vi "Agilent ENA Series Receiver Measurements.vi"() -> ()   [LabVIEW 2020]
doc: "Illustrates typical measuring task for a network analyzer by setting receiver leveling. It measures a band-pass filter (center frequency: 947.5 MHz), and calculates and displays its bandwidth, insertion loss, and so on.\n\nNote:\n(1) For this function you must set DUT on instrument.\n(2) Valid for E5072A only."
uses:
  <instrlib>/Agilent ENA Series/Agilent ENA Series.lvlib
panel:
  in  "Safe Mode Maximum Power Level (30)":dbl=30.0
  in  "Safe Mode Minimum Power Level (-200)":dbl=-200.0
  in  "Tolerance Level (5)":dbl=5.0
  in  "Power Level Offset (0)":dbl
  in  "Port ( 1)":i32=1
  in  "Channel (1)":i32=1
  in  "Enable Safe Mode (T: Enabled)":bool=TRUE
  in  "Enable Receiver Leveling (T: Enabled)":bool=TRUE
  in  "Reset? (T: Yes)":bool=TRUE
  in  "ID Query? (T: Yes)":bool=TRUE
  out "High":dbl
  out "Low":dbl
  out "Center Frequency":dbl format="%^.2e"
  out "Q Value":dbl format="%^.2e"
  out "Loss":dbl format="%^.2e"
  out "Bandwidth":dbl format="%^.2e"
  in  "VISA resource name":refnum<visa-resource-name>
  # "(c) 2014-2021 National Instruments.  ALL RIGHTS RESERVED."
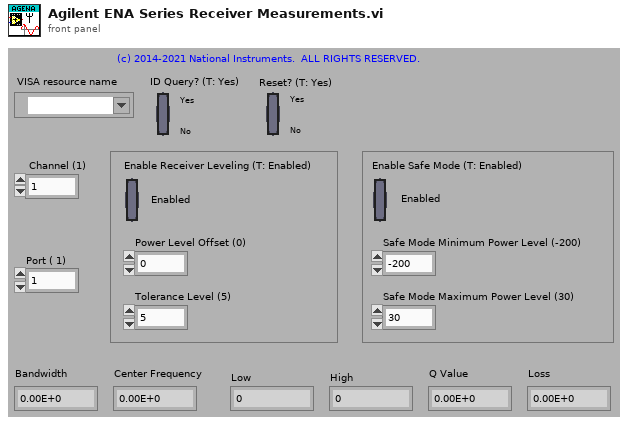
[diagram p1: front panel]
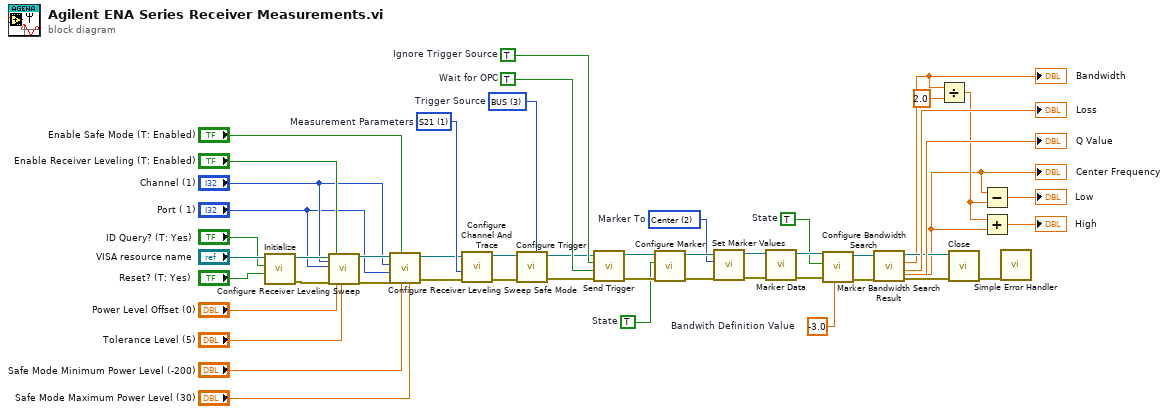
[diagram p0: block diagram]
diagram:
  w17 = u16 1 items=["S11", "S21", "S31", "S41", "S12", "S22", "S32", "S42", "S13", "S23", "S33", "S43", "S14", "S24", "S34", "S44", "A", "B", "C", "D", "R1", "R2", "R3", "R4"]  # Measurement Parameters
  w36 = -3.0  # Bandwith Definition Value
  w37 = TRUE  # State
  w42 = u16 2 items=["Start", "Stop", "Center", "Reference", "Electrical Delay"]  # Marker To
  w45 = TRUE  # State
  w48 = TRUE  # Wait for OPC
  w49 = TRUE  # Ignore Trigger Source
  w50 = u16 3 items=["Internal", "External", "Manual", "BUS"]  # Trigger Source
  n1 = call <instrlib>:"Initialize.vi"("Reset? (T: Yes)"="Reset? (T: Yes)", "ID Query? (T: Yes)"="ID Query? (T: Yes)", "VISA resource name"="VISA resource name") -> ("error out"=w15:errorcluster, "VISA resource name out"=w16:refnum<visa-resource-name>)  [unwired: 7 in]
  n2 = call <instrlib>:"Configure Receiver Leveling Sweep.vi"("VISA resource name"=w16, "Channel (1)"="Channel (1)", "Port ( 1)"="Port ( 1)", "error in (no error)"=w15, "Enable Receiver Leveling (F: Disabled)"="Enable Receiver Leveling (T: Enabled)", "Power Level Offset (0)"="Power Level Offset (0)", "Tolerance Level (5)"="Tolerance Level (5)") -> ("VISA resource name out"=w10:refnum<visa-resource-name>, "error out"=w9:errorcluster)  [unwired: 11 in]
  n3 = call <instrlib>:"Configure Receiver Leveling Sweep Safe Mode.vi"("Safe Mode Maximum Power Level (30)"="Safe Mode Maximum Power Level (30)", "Safe Mode Minimum Power Level (-200)"="Safe Mode Minimum Power Level (-200)", "Enable Safe Mode (F: Disabled)"="Enable Safe Mode (T: Enabled)", "error in (no error)"=w9, "Port ( 1)"="Port ( 1)", "Channel (1)"="Channel (1)", "VISA resource name"=w10) -> ("error out"=w13:errorcluster, "VISA resource name out"=w14:refnum<visa-resource-name>)  [unwired: 3 in]
  n4 = call <instrlib>:"Configure Channel And Trace.vi"("error in (no error)"=w13, "Measurement Parameters (0: S11)"=w17, "VISA resource name"=w14) -> ("error out"=w11:errorcluster, "VISA resource name out"=w12:refnum<visa-resource-name>)  [unwired: 7 in]
  n5 = call <instrlib>:"Configure Trigger.vi"("Trigger Source (0: Internal)"=w50, "error in (no error)"=w11, "VISA resource name"=w12) -> ("error out"=w18:errorcluster, "VISA resource name out"=w19:refnum<visa-resource-name>)  [unwired: 7 in]
  n6 = call <instrlib>:"Send Trigger.vi"("error in (no error)"=w18, "Wait for OPC (F: Do not Wait)"=w48, "Ignore Trigger Source (F: Do not Ignore)"=w49, "VISA resource name"=w19) -> ("error out"=w46:errorcluster, "VISA resource name out"=w47:refnum<visa-resource-name>)  [unwired: 6 in]
  n7 = call <instrlib>:"Configure Marker.vi"("error in (no error)"=w46, "Marker State (F: Disabled)"=w45, "VISA resource name"=w47) -> ("error out"=w43:errorcluster, "VISA resource name out"=w44:refnum<visa-resource-name>)  [unwired: 7 in]
  n8 = call <instrlib>:"Set Marker Values.vi"("error in (no error)"=w43, "Marker To (0: Start)"=w42, "VISA resource name"=w44) -> ("error out"=w40:errorcluster, "VISA resource name out"=w41:refnum<visa-resource-name>)  [unwired: 7 in]
  n9 = call <instrlib>:"Marker Data.vi"("error in (no error)"=w40, "VISA resource name"=w41) -> ("error out"=w38:errorcluster, "VISA resource name out"=w39:refnum<visa-resource-name>)  [unwired: 5 in, 3 out]
  n10 = call <instrlib>:"Configure Bandwidth Search.vi"("Bandwidth Definition Value (-3.0)"=w36, "error in (no error)"=w38, "Result Display State (F: Disable)"=w37, "VISA resource name"=w39) -> ("error out"=w34:errorcluster, "VISA resource name out"=w35:refnum<visa-resource-name>)  [unwired: 6 in]
  n11 = call <instrlib>:"Marker Bandwidth Search Result.vi"("error in (no error)"=w34, "VISA resource name"=w35) -> ("error out"=w30:errorcluster, "Loss"=→"Loss":dbl, "Bandwidth"=w29:dbl, "VISA resource name out"=w31:refnum<visa-resource-name>, "Q Value"=→"Q Value":dbl, "Center Frequency"=w25:dbl)  [unwired: 4 in]
  "Bandwidth" <- w29
  "Center Frequency" <- w25
  n12 = Divide(x=w29, y=2.0) -> (x/y=w26:dbl)
  n13 = call <instrlib>:"Close.vi"("error in (no error)"=w30, "VISA resource name"=w31) -> ("error out"=w23:errorcluster)  [unwired: 9 in]
  n14 = Subtract(x=w25, y=w26) -> (x-y=→"Low":dbl)
  n15 = Add(x=w26, y=w25) -> (x+y=→"High":dbl)
  n16 = call <vilib>:"Simple Error Handler.vi"("error in (no error)"=w23) -> ()  [unwired: 4 in, 5 out]
